vi "Set Changed Event.vi"(10 "Changed Event":refnum<user-event>, 11 "ColumnPanel in":refnum<class "ColumnPanel.lvclass">) -> (3 "ColumnPanel out":refnum<class "ColumnPanel.lvclass">)   [LabVIEW 2020, in "Conditum-Tools.lvlib" / "ColumnPanel.lvclass"]
uses:
  ColumnPanel.lvclass
  ColumnPanel.lvclass/ColumnPanel.ctl
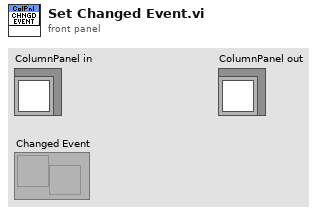
[diagram p1: front panel]
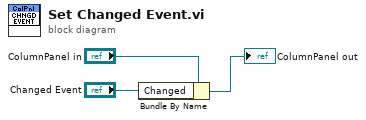
[diagram p0: block diagram]
diagram:
  n1 = Bundle By Name(cluster="ColumnPanel in", "Changed"="Changed Event") -> (→"ColumnPanel out":refnum<class "ColumnPanel.lvclass">)
